vi "压力稳定状态.vi"(3 "error in (no error) 2":errorcluster caption="错误输入（无错误）", 5 "VISA resource name":refnum<visa-resource-name> caption="VISA资源名称") -> (0 "错误输出":errorcluster, 1 "状态(1稳定)":string, 2 "VISA资源名称输出":refnum<visa-resource-name>)   [LabVIEW 2017]
panel:
  in  "等待时间（毫秒）":u32=100
  in  "写":bool=TRUE
  in  "指令":string="OUTPut:STABle?"
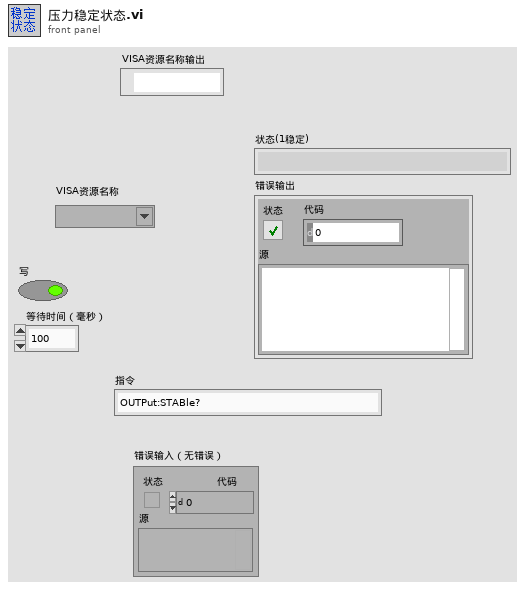
[diagram p1: front panel]
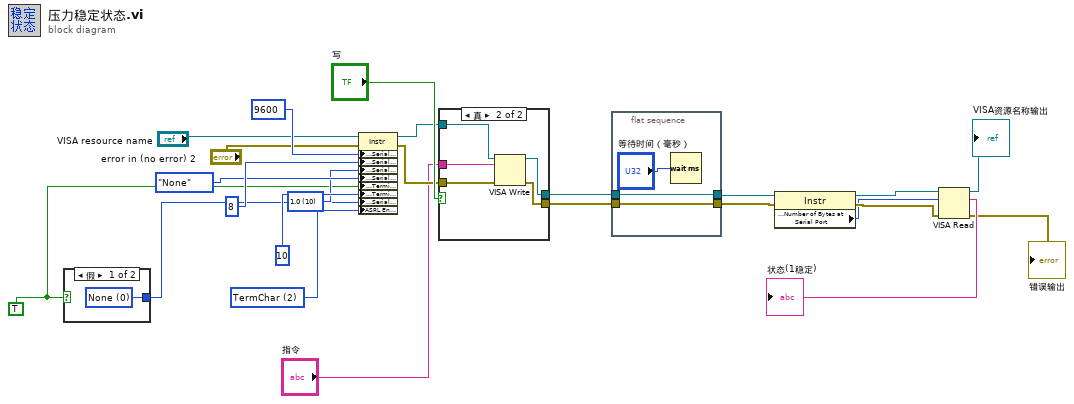
[diagram p0: block diagram]
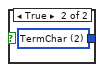
[diagram p2: hidden frame]
diagram:
  w7 = TRUE ("Enable Termination\nChar (T) 2")
  w6 = u16 2 items=["None", "Last Bit", "TermChar", "Break"] ("Serial Settings:End Mode for Writes")
  w9 = u16 10 items=["1.0"=10, "1.5"=15, "2.0"=20] ("stop bits (10: 1 bit)")
  n1 = case shown="假" w7 {
    tunnel: [w25 w26] -> w8
    frame False {
      w25 = u16 0 items=["None", "LastBit", "TermChar"] ("Serial Settings:Serial End Mode for Reads")
    }
    frame True {
      w26 = u16 2 items=["None", "LastBit", "TermChar"] ("Serial Settings:Serial End Mode for Reads")
    }
  }
  n2 = property class="Instr"(reference="VISA resource name", error in="error in (no error) 2", "Serial Settings:Serial Baud Rate"=u32 9600 ("baud rate (9600)"), "Serial Settings:Serial Data Bits"=u16 8 ("data bits (8)"), "Serial Settings:Serial Stop Bits"=w9, "Serial Settings:Serial Parity"=enum16{"None", "Odd", "Even", "Mark", "Space"}."None" ("parity (0:none)"), "Message Based Settings:Termination Character Enable"=w7, "Message Based Settings:Termination Character"=u8 10 ("termination char\n(0xA = '\\n' = LF)"), "Serial Settings:Serial End Mode for Reads"=w8, "ASRL End Out"=w6) -> (reference out=w5:refnum<visa-resource-name>, error out=w4:errorcluster)
  n3 = case shown="真" "写" {
    tunnel: "指令" -> [_ w33]
    tunnel: [w28 w32] -> w23
    tunnel: [w27 w31] -> w22
    tunnel: w5 -> [w27 w30]
    tunnel: w4 -> [w28 w29]
    frame False {
    }
    frame True {
      n4 = VISA Write(VISA resource name=w30, write buffer=w33, error in (no error)=w29) -> (VISA resource name out=w31:refnum<visa-resource-name>, error out=w32:errorcluster)  [unwired: 1 out]
    }
  }
  n5 = flat-sequence {
    tunnel: w23 -> [w34]
    tunnel: w22 -> [w35]
    tunnel: [w35] -> w19
    tunnel: [w34] -> w18
    frame #0 {
      n6 = Wait (ms)(milliseconds to wait="等待时间（毫秒）") -> ()  [unwired: 1 out]
    }
  }
  n7 = property class="Instr"(reference=w19, error in=w18) -> (reference out=w21:refnum<visa-resource-name>, error out=w20:errorcluster, "Serial Settings:Number of Bytes at Serial Port"=w17:u32)
  n8 = VISA Read(VISA resource name=w21, byte count=w17, error in (no error)=w20) -> (VISA resource name out=→"VISA资源名称输出":refnum<visa-resource-name>, read buffer=→"状态(1稳定)":string, error out=→"错误输出":errorcluster)  [unwired: 1 out]
